vi "I2C Read.vi"(9 "pdata":string, 10 "intAddress":u8, 11 "deviceID":u8) -> (1 "pdata out":string, 3 "function return":u32)   [LabVIEW 2018, in "AndorSDK.lvlib"]
doc: "EXPNETTYPE unsigned int WINAPI I2CRead(BYTE deviceID, BYTE intAddress, BYTE * pdata);"
uses:
  AndorSDK.lvlib
  ATMCD32D.dll
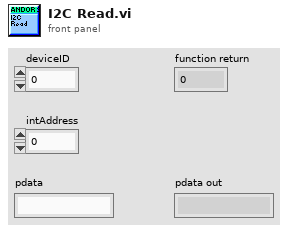
[diagram p1: front panel]
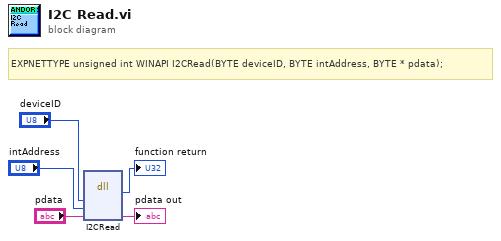
[diagram p0: block diagram]
diagram:
  # "EXPNETTYPE unsigned int WINAPI I2CRead(BYTE deviceID, BYTE intAddress, BYTE * pdata);"
  n1 = dll-call lib="PTH2babs E\nPersönliches02 - Arbeit03-HiwijobsLabviewCodelibANDOR\tAndor SDK\nATMCD32D.*" fn="I2CRead"("deviceID"="deviceID", "intAddress"="intAddress", "pdata"="pdata") -> (→"function return":u32, "pdata"=→"pdata out":string)  [unwired: 5 in, 2 out]
